vi "Set Trigger Levelm V.vi"(8 "error in (no error)":errorcluster, 10 "sense_mv":i32, 11 "level_mv":i32) -> (0 "error out":errorcluster)   [LabVIEW 2021, in "vmmso.lvlib"]
doc: "DLL_API void WINAPI SetTriggerLevelmV(int level_mv, int sense_mv);"
uses:
  vmmso.lvlib
  vmmso.dll
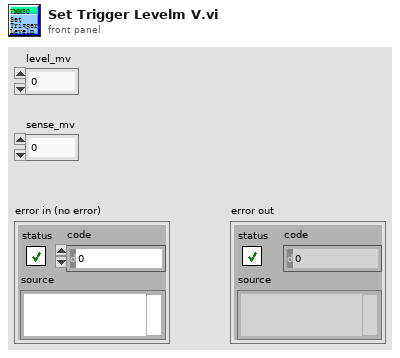
[diagram p1: front panel]
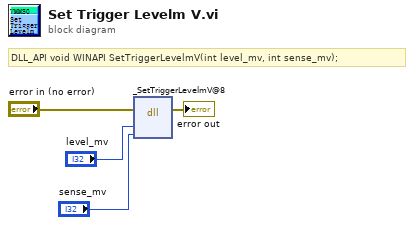
[diagram p0: block diagram]
diagram:
  # "DLL_API void WINAPI SetTriggerLevelmV(int level_mv, int sense_mv);"
  n1 = dll-call lib="O:/MSO/library/demo-Labview/vmmso/vmmso.*" fn="_SetTriggerLevelmV@8"(error in="error in (no error)", "level_mv"="level_mv", "sense_mv"="sense_mv") -> (error out=→"error out":errorcluster)  [unwired: 5 in, 1 out]
